vi "Target Centralization.vi"(0 "Camera Angle":dbl=35.25, 1 "Target Limit":dbl=0.03, 2 "Servo Angle in":dbl, 3 "Camera Axis Position":dbl, 4 "Servo Horizontal Angle":dbl=22.0, 5 "Distance From Target":dbl) -> (6 "Servo Angle out":dbl)   [LabVIEW 2012]
panel:
  in  "Camera view angle":dbl[](array[numeric])=[48.0, 43.5]
  in  "Camera Type":enum16{"206", "1011"}(ring)=enum."1011"
  # "axis 206"
  # "axis 1011"
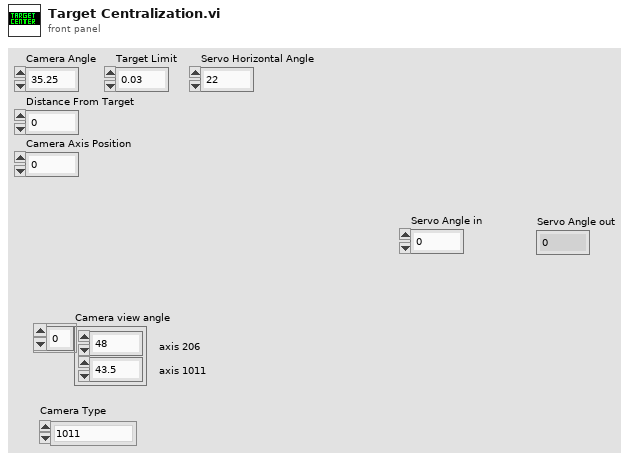
[diagram p1: front panel]
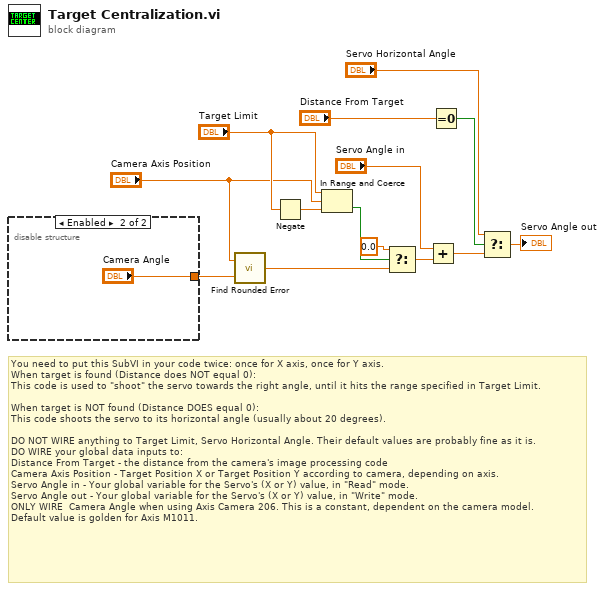
[diagram p0: block diagram]
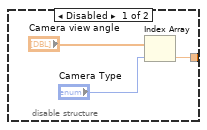
[diagram p2: hidden frame]
diagram:
  # "You need to put this SubVI in your code twice: once for X axis, once for Y axis.\nWhen target is found (Distance does NOT equal 0):\nThis code is used to \"shoot\" the servo towards the right angle, until it hits the range specified in Target Limit.\n\nWhen target is NOT found (Distance DOES equal 0):\nThis code shoots the servo to its horizontal angle (usually about 20 degrees).\n\nDO NOT WIRE anything to Target Limit, Servo Horizontal Angle. Their default values are probably fine as it is.\nDO WIRE your global data inputs to:\nDistance From Target - the distance from the camera's image processing code\nCamera Axis Position - Target Position X or Target Position Y according to camera, depending on axis.\nServo Angle in - Your global variable for the Servo's (X or Y) value, in \"Read\" mode.\nServo Angle out - Your global variable for the Servo's (X or Y) value, in \"Write\" mode.\nONLY WIRE  Camera Angle when using Axis Camera 206. This is a constant, dependent on the camera model.\nDefault value is golden for Axis M1011."
  n1 = disable-structure shown="Enabled" {
    disable-tunnel: [w15 "Camera Angle"] -> w1
    frame Disabled {
      n2 = Index Array(array="Camera view angle", index="Camera Type") -> (element=w15:dbl)
    }
    frame Enabled {
    }
  }
  n3 = call "Find Rounded Error.vi"("Camera Angle"=w1, "Camera Axis Position"="Camera Axis Position") -> ("Rounded Error"=w2:dbl)
  n4 = Negate(x="Target Limit") -> (-x=w12:dbl)
  n5 = In Range and Coerce(upper limit="Target Limit", x="Camera Axis Position", lower limit=w12) -> (In Range?=w10:bool)  [unwired: 1 out]
  n6 = Select(t=0.0, s=w10, f=w2) -> (s? t:f=w9:dbl)
  n7 = Add(x="Servo Angle in", y=w9) -> (x+y=w5:dbl)
  n8 = Equal To 0?(x="Distance From Target") -> (x = 0?=w7:bool)
  n9 = Select(t="Servo Horizontal Angle", s=w7, f=w5) -> (s? t:f=→"Servo Angle out":dbl)
